vi "Create MeasLink APIs.vi"(0 "Logic VI Ref":refnum<vi>, 11 "error in (no error)":errorcluster) -> (4 "Logic VI Out":refnum<vi>, 6 "SubVI Refrences":refnum<vi>[](array[refnum]), 15 "error out":errorcluster)   [LabVIEW 2021, in "Converter.lvlib"]
uses:
  Converter.lvlib
  <vilib>/Utility/miscctls.llb/LVPointTypeDef.ctl
  Path Functions/Path Functions.lvlib
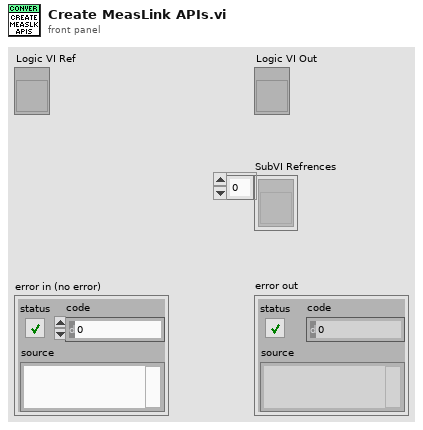
[diagram p1: front panel]
types:
  T1 = typedef "LVPointTypeDef.ctl" = cluster{"Horizontal":i16, "Vertical":i16}
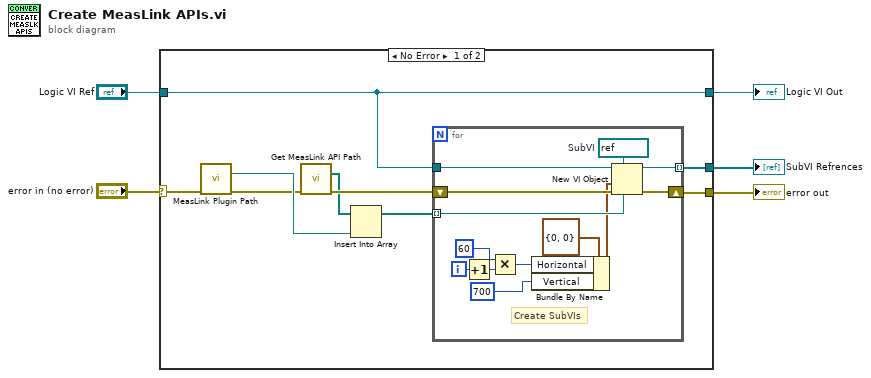
[diagram p0: block diagram]
diagram:
  n1 = case shown="No Error" "error in (no error)" {
    selector: "error in (no error)" -> [w8 w28]
    tunnel: [w11 _] -> w5
    tunnel: [w9 w28] -> w4
    tunnel: "Logic VI Ref" -> [w6 w29]
    tunnel: [w6 w29] -> w1
    frame No Error {
      n2 = call "MeasLink Plugin Path.vi"("error in (no error)"=w8) -> ("Wrapper Path"=w14:path, "error out"=w7:errorcluster)  [unwired: 2 in, 11 out]
      n3 = call "Get MeasLink API Path.vi"("error in (no error)"=w7) -> ("MeasLink API Paths"=w12:path[], "error out"=w13:errorcluster)  [unwired: 13 in]
      n4 = Insert Into Array(array=w12, new element=w14) -> (w10:path[])  [unwired: 1 in]
      n5 = for {
        tunnel: w10 -> [w26] mode=indexing
        tunnel: w6 -> [w25]
        tunnel: [w20] -> w11 mode=indexing
        shift-right: [w21] -> w9
        shift-left: w13 -> [w27]
        i -> [w18]
        w24 = refnum<vi> refnum  # SubVI
        # "Create SubVIs"
        n6 = Increment(x=w18) -> (x+1=w15:i32)
        n7 = Multiply(x=i16 60 ("Vertical"), y=w15) -> (x*y=w17:i32)
        n8 = Bundle By Name(cluster=T1 {"Horizontal"=0, "Vertical"=0} ("location"), "Horizontal"=w17, "Vertical"=i16 700) -> (w22:T1)
        n9 = New VI Object(vi object class=w24, owner refnum=w25, position/next to=w22, 6:w26, 8:w27) -> (object refnum=w20:refnum<vi>, 0:w21:errorcluster)  [unwired: 3 in]
      }
    }
    frame Error {
    }
  }
  "SubVI Refrences" <- w5
  "error out" <- w4
  "Logic VI Out" <- w1
